vi "Generating Continuous Digital Pulse Train with a Variable Frequency - LV2012 NI Verified.vi"() -> ()   [LabVIEW 2018]
doc: "I. Description:\nThis example demonstrates how to generate a continuous digital pulse train from a Counter Output Channel. The Frequency, Duty Cycle, and Idle State are all configurable. \n\nThis example shows how to configure the pulse in terms of Frequency/Duty Cycle, but can easily be modified to generate a pulse in terms of Time or Ticks.\n\nII. Instructions for Running:\n1. Select the Physical Channel which corresponds to the counter you want to output your signal to on the DAQ device.\n2. Enter the Frequency and Duty Cycle to define the pulse parameters. You can also change the Idle State to determine the beginning and end states of the output. If the Idle State is High, the generation will use inverted logic. Additionally, you can set the Initial Delay (in seconds) which will delay the beginning of the pulse train from the start call; this is currently wired to 0.0 on the diagram. \nNote: Use the Measure Period example to verify you are outputting the pulse train on the DAQ device.\n\nIII. Block Diagram Steps:\n1. Create a Counter Output channel to produce a Pulse in terms of Frequency. If the Idle State of the pulse is set to low, the state of the line will begin low and remain low after the generation is stopped.\n2. Use the DAQmx Timing VI (Implicit) to configure the duration of the pulse generation.\n3. Call the Start VI to arm the counter and begin the pulse train generation.\n4. Loop continuously until the user presses the Stop button. Check for errors every 100 ms using the Is Task Done? VI\n5. Call the Clear Task VI to clear the Task.\n\nIV. I/O Connections Overview:\nThe counter will output the pulse train on the output terminal of the counter specified in the Physical Channel I/O control. \n\nIn this example the output will be sent to the default output terminal on ctr0.\n\nFor more information on the default counter input and output terminals for your device, open the NI-DAQmx Help, and refer to Counter Signal Connections found under the Device Considerations book in the table of contents."
uses:
  <vilib>/Utility/error.llb/DialogType.ctl
  <vilib>/DAQmx/create/channels.llb/DAQmx Create Channel (CO-Pulse Generation-Frequency).vi
  <vilib>/DAQmx/configure/timing.llb/DAQmx Timing (Implicit).vi
  <resource>/objmgr/daqmx.rc
panel:
  in  "Duty Cycle":dbl=0.5 min=0.0 max=1.0 format="%0.2f"
  in  "Frequency":dbl=1.0 caption="Frequency (Hz)" format="%0.2f"
  in  "Idle State":i32(ring)=10214 items=["High"=10192, "Low"=10214]
  in  "Counter(s)":tag="Dev1/ctr0"
  in  "stop":bool
  # "Overview: Demonstrates how to generate a continuous pulse train with\nconfigurable frequency input\nRequirement: LabVIEW Full Development System\nInstructions:\n1. Set the physical channel of the counter\n2. (Optional) Define the rest of the parameters as needed\n3. Run the VI"
  # "For instructions, select Help>>Show Context Help"
  # "Channel Parameters"
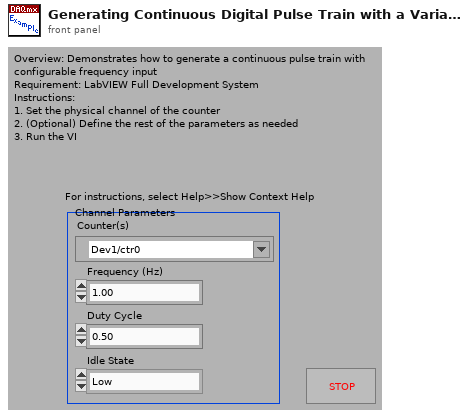
[diagram p1: front panel]
types:
  T1 = typedef "DialogType.ctl" = u16
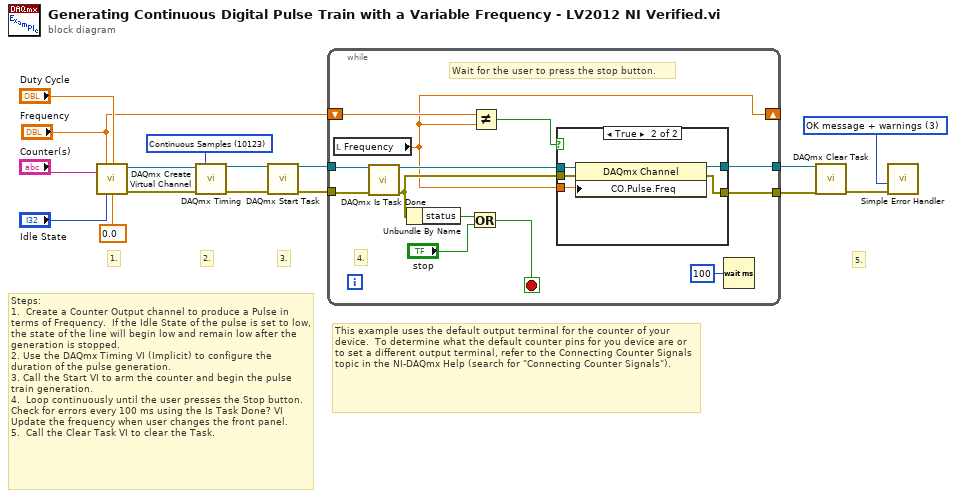
[diagram p0: block diagram]
diagram:
  w2 = T1 3 items=["no dialog", "OK message", "continue or stop message", "OK message + warnings", "continue/stop + warnings"] ("type of dialog (OK msg:1)")
  w8 = 10123 items=["Finite Samples"=10178, "Continuous Samples"=10123] ("sample mode")
  # "This example uses the default output terminal for the counter of your device.  To determine what the default counter pins for you device are or to set a different output terminal, refer to the Connecting Counter Signals topic in the NI-DAQmx Help (search for \"Connecting Counter Signals\")."
  # "Steps: \n1.  Create a Counter Output channel to produce a Pulse in terms of Frequency.  If the Idle State of the pulse is set to low, the state of the line will begin low and remain low after the generation is stopped.\n2. Use the DAQmx Timing VI (Implicit) to configure the duration of the pulse generation.\n3. Call the Start VI to arm the counter and begin the pulse train generation.\n4.  Loop continuously until the user presses the Stop button. Check for errors every 100 ms using the Is Task Done? VI\nUpdate the frequency when user changes the front panel.\n5.  Call the Clear Task VI to clear the Task."
  # "5."
  # "3."
  # "2."
  # "1."
  n1 = call-poly <vilib>:"DAQmx Create Virtual Channel.vi"("frequency"="Frequency", "duty cycle"="Duty Cycle", "counter"="Counter(s)", "idle state"="Idle State", "initial delay"=0.0) -> ("task out"=w13:refnum<k21>, "error out"=w16:errorcluster)  [unwired: 9 in]
  n2 = call-poly <vilib>:"DAQmx Timing.vi"("task/channels in"=w13, "sample mode"=w8, "error in"=w16) -> ("task out"=w9:refnum<k21>, "error out"=w10:errorcluster)  [unwired: 11 in]
  n3 = call <vilib>:"DAQmx Start Task.vi"("task/channels in"=w9, "error in"=w10) -> ("task out"=w12:refnum<k21>, "error out"=w15:errorcluster)  [unwired: 12 in]
  n4 = while {
    tunnel: w15 -> [w28]
    tunnel: w12 -> [w29]
    tunnel: [w23] -> w11
    tunnel: [w19] -> w3
    shift-right: [w18] -> _
    shift-left: "Frequency" -> [w21]
    stop <- w27 stop-if-true
    # "Wait for the user to press the stop button."
    # "4."
    n5 = local read "Frequency"() -> (w18:dbl)
    n6 = call <vilib>:"DAQmx Is Task Done.vi"("task/channels in"=w29, "error in"=w28) -> ("task out"=w24:refnum<k21>, "error out"=w22:errorcluster)  [unwired: 11 in, 1 out]
    n7 = Unbundle By Name(w22) -> ("status"=w26:bool)
    n8 = Or(x=w26, y="stop") -> (x .or. y?=w27:bool)
    n9 = Not Equal?(x=w21, y=w18) -> (x != y?=w20:bool)
    n10 = case shown="True" w20 {
      tunnel: w24 -> [w31 w36]
      tunnel: w18 -> [_ w35]
      tunnel: [w31 w34] -> w23
      tunnel: w22 -> [w30 w33]
      tunnel: [w30 w32] -> w19
      frame False {
      }
      frame True {
        n11 = property class="DAQmx Channel"(reference=w36, error in=w33, "CO.Pulse.Freq"=w35) -> (reference out=w34:refnum<k21>, error out=w32:errorcluster)
      }
    }
    n12 = Wait (ms)(milliseconds to wait=u32 100) -> ()  [unwired: 1 out]
  }
  n13 = call <vilib>:"DAQmx Clear Task.vi"("task in"=w11, "error in"=w3) -> ("error out"=w14:errorcluster)  [unwired: 13 in]
  n14 = call <vilib>:"Simple Error Handler.vi"("type of dialog (OK msg:1)"=w2, "error in (no error)"=w14) -> ()  [unwired: 3 in, 5 out]
